vi "Control of Actuator Gait Retraining Actuator Based on IMU Signals.vi"() -> ()   [LabVIEW 2018]
uses:
  <vilib>/Platform/TimedLoop/XDataNode/timing_clust.ctl
  <vilib>/Platform/TimedLoop/XDataNode/nitl_modes.ctl
  <vilib>/Platform/TimedLoop/XDataNode/wakeup.ctl
  <vilib>/DAQmx/write.llb/DAQmx Write (Digital Bool 1Line 1Point).vi
  <vilib>/DAQmx/read.llb/DAQmx Read (Digital Bool 1Line 1Point).vi
  <vilib>/Utility/file.llb/Read Delimited Spreadsheet (DBL).vi
  <vilib>/DAQmx/create/channels.llb/DAQmx Create Channel (DI-Digital Input).vi
  <vilib>/DAQmx/miscellaneous.llb/DAQmx Fill In Error Info.vi
  <vilib>/DAQmx/create/channels.llb/DAQmx Create Channel (DO-Digital Output).vi
  <vilib>/platform/TimedLoop/XDataNode/XDataNode.xnode
  <vilib>/Platform/TimedLoop/XDataNode/XDNodeRunTimeDep.lvlib
  <vilib>/Analysis/NI_AALBase.lvlib
panel:
  out "Stride Pert R":dbl
  out "Stride R T":dbl
  in  "Delay Decimal":dbl
  out "LATENCY MS":dbl
  out "Combined Results":dbl[][][](array[numeric])
  out "INIT END":dbl[][](array[numeric])
  out "Go Right":bool
  out "Go Left":bool
  out "Latency ms":dbl
  out "Stride Pert L":dbl
  out "Stride L T":dbl
  out "EXTEND":bool=TRUE
  out "RETRACT":bool=TRUE
  out "REST":bool=TRUE
  out "MS Start":u32
  out "Boolean":bool=TRUE
  out "Right Stop":dbl
  out "Right Start":dbl
  out "Left Stop":dbl
  out "Left Start":dbl
  out "End L":dbl[](array[numeric])
  out "Init L":dbl[](array[numeric])
  out "End R":dbl[](array[numeric])
  out "Init R":dbl[](array[numeric])
  out "Peaks L":dbl[](array[numeric])
  out "Peaks R":dbl[](array[numeric])
  out "TO R":dbl[](array[numeric])
  out "TO L":dbl[](array[numeric])
  out "Fire Right":bool=TRUE
  out "Fire Left":bool=TRUE
  out "Loop It":i32
  out "x-y":i32
  out "Mu L":dbl
  out "Mu R":dbl
  out "Sig L":dbl format="%0.2f"
  out "Sig R":dbl format="%0.2f"
  out "L Buffer":dbl[](array[numeric])
  out "R Buffer":dbl[](array[numeric])
  out "L Data":dbl[](array[numeric])
  out "R Data":dbl[](array[numeric])
  out "Length L":i32
  out "Swing L":bool
  out "Swing R":bool
  out "Peaked L":bool
  out "Peaked R":bool
  out "Count L":i32=100
  out "Count R":i32=100
  out "Peak Num L":i32=100
  out "Peak Num R":i32=100
  out "TO Num L":i32=100
  out "TO Num R":i32=100
  out "Neg L":i32=100
  out "Neg R":i32=100
  out "Stride L":i32=100
  out "Stride R":i32=100
  out "Stance L":bool
  out "Stance R":bool
  out "Iteration":i32
  out "End":bool=TRUE
  in  "Pressure (Bar)":dbl
  in  "Pert Decimal":dbl
  out "Count":i32
  out "SW2 Off":dbl
  out "transposed array":dbl[][](array[numeric])
  out "Results":dbl[][](array[numeric])
  in  "Extend Time":dbl
  out "Extend Limit":dbl
  out "SW2 Pressed":bool
  in  "V Ext":bool
  in  "V Ret":bool
  out "SW1 Off":dbl
  out "SW1 Pressed":bool
  in  "Extend":bool
  in  "Retract":bool
  out "SW2":bool
  out "SW1":bool
  out "ms passed":dbl
  in  "STOP":bool
  # "May need to switch off if not working"
  # "Percentage of\nGait Cycle"
  # "Percentage of \nGait Cycle"
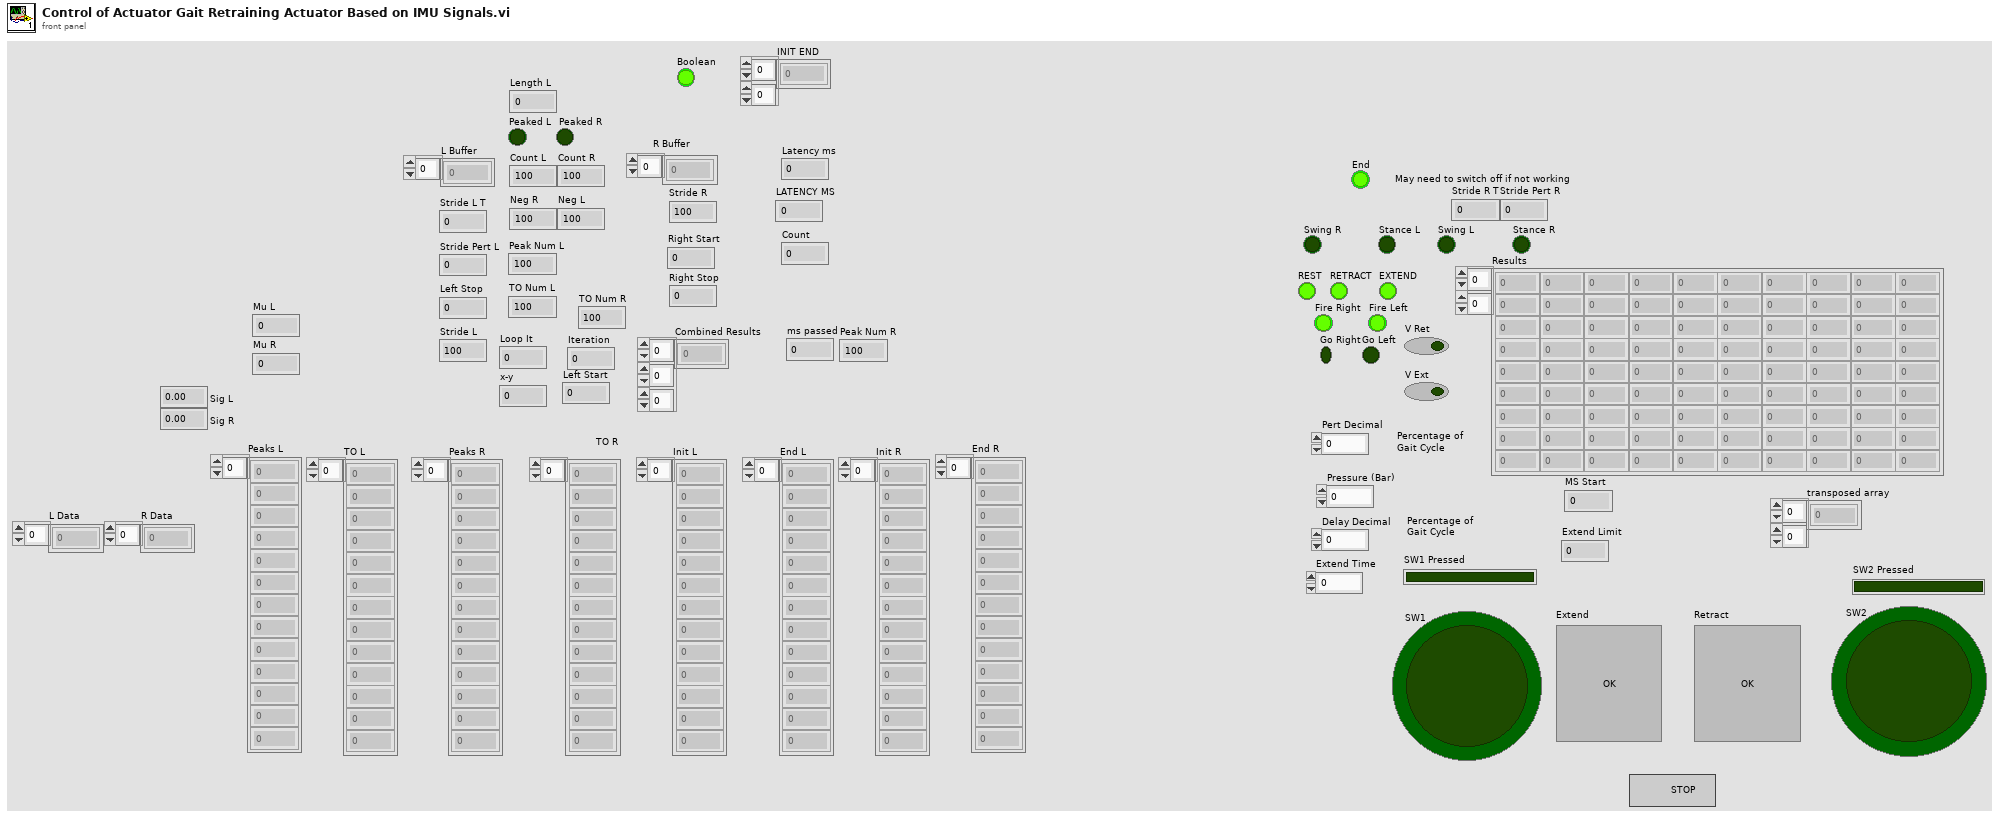
[diagram p1: front panel]
types:
  T1 = typedef "XDNodeRunTimeDep.lvlib/timing_clust.ctl" = cluster{"Expected End [f-1]":u64, "Actual End [f-1]":u64, "Finished Late? [f-1]":bool, "Expected End [i-1]":u64, "Actual End [i-1]":u64, "Finished Late? [i-1]":bool, "Expected Start [i]":u64, "Actual Start [i]":u64, "Expected Start [f]":u64, "Actual Start [f]":u64, "Source Name":string, "Structure Name":string, "Period":i64, "Deadline":i64, "Offset":i64, "Start":i64, "Priority":i32, "Timeout":i32, "Mode":T2, "Wakeup Reason":T3, "Error":errorcluster, "Source Type":string, "Secondary Source Type":string, "Global End Time":u64, "Global Start Time":u64, "Frame Duration":u64, "Iteration Duration":u64, "Assigned CPU":i32, "I/O Scan Engine Mode":u32}
  T2 = typedef "XDNodeRunTimeDep.lvlib/nitl_modes.ctl" = enum32{"No Change", "Process missed periods, maintain original phase", "Discard missed periods, maintain original phase", "Process missed periods, ignore original phase", "Discard missed periods, ignore original phase"}
  T3 = typedef "XDNodeRunTimeDep.lvlib/wakeup.ctl" = enum32{"Normal", "Aborted", "Asynchronous wakeup", "Timing source error", "Timed loop error", "Timeout"}
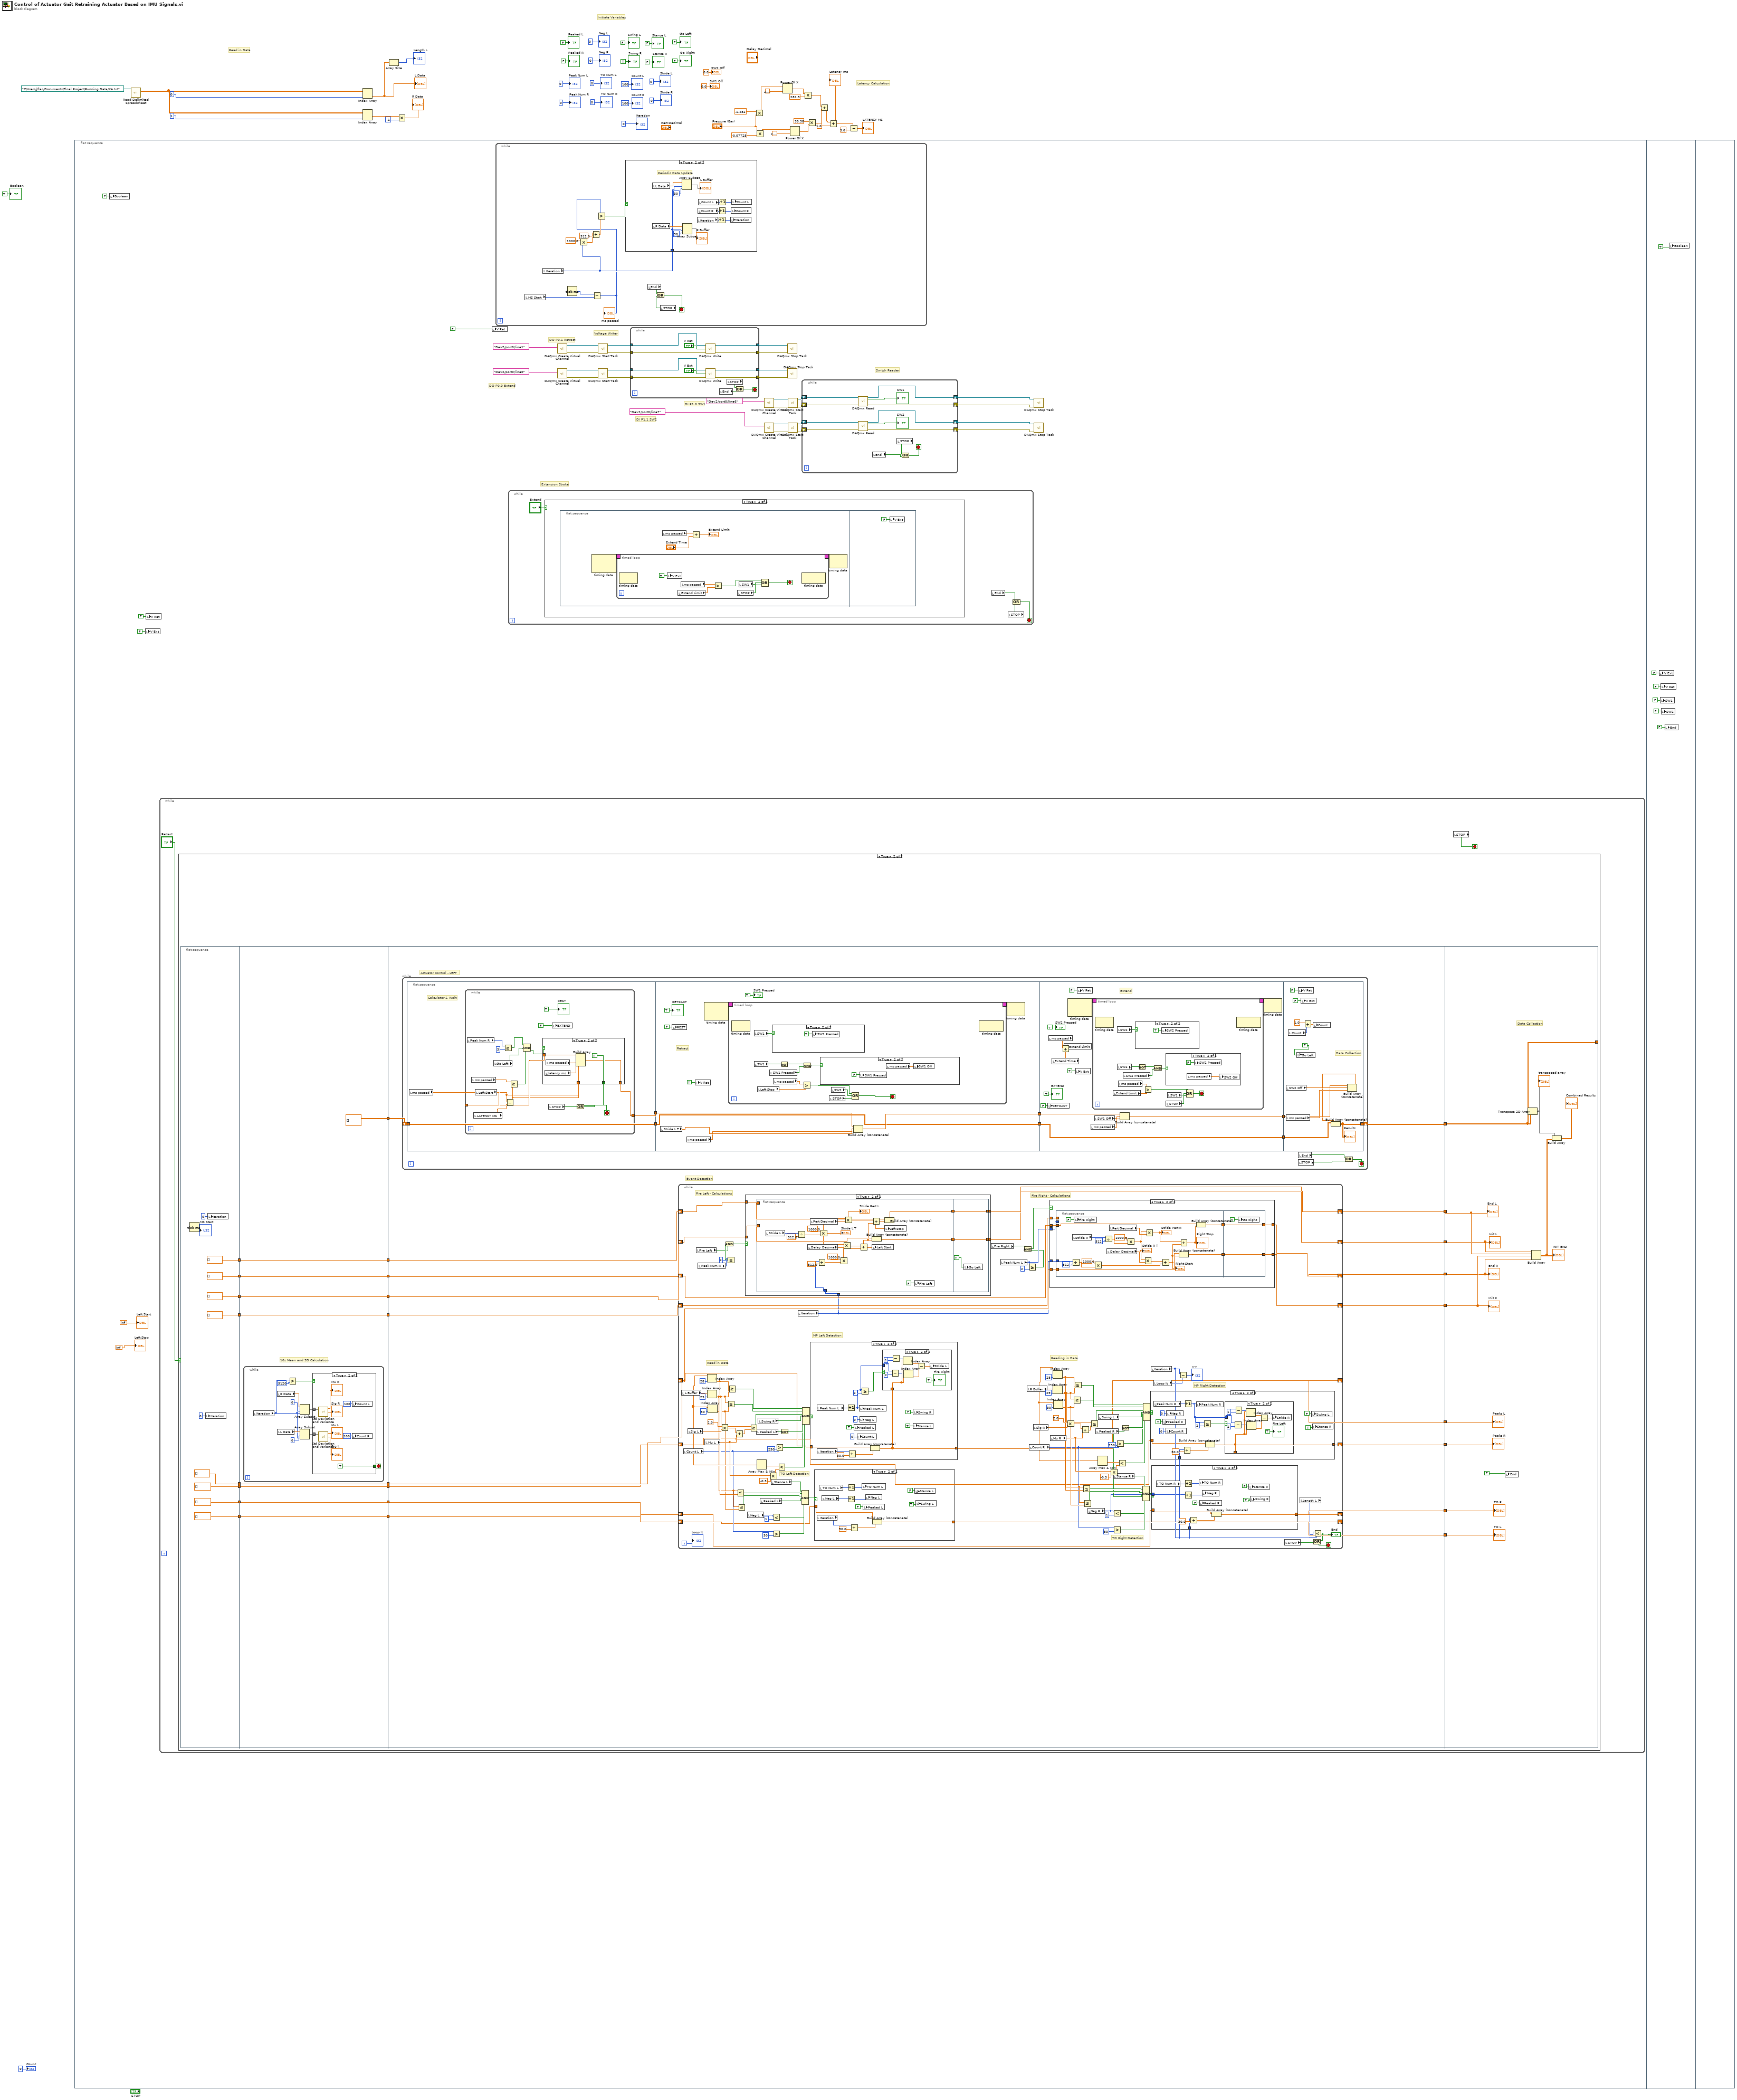
[diagram p0: block diagram]
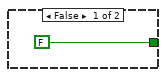
[diagram p4: hidden frame]
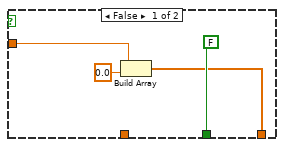
[diagram p5: hidden frame]
diagram:
  # "Latency Calculation"
  # "Initiate Variables"
  # "Read in Data"
  n1 = flat-sequence {
    frame #0 {
      # "Extension Stroke"
      # "Switch Reader"
      # "Voltage Writer"
      # "DO P0.1 Retract"
      # "DO P0.0 Extend"
      # "DI P1.1 SW2"
      # "DI P1.0 SW1"
      n2 = local write "Boolean"(FALSE ("Boolean")) -> ()
      n3 = local write "V Ext"(FALSE ("V Ext")) -> ()
      n4 = local write "V Ret"(FALSE ("V Ret")) -> ()
      n5 = while {
        stop <- w120 stop-if-true
        n6 = case shown="True" "Retract" {
          frame False {
          }
          frame True {
            n7 = flat-sequence {
              tunnel: [dbl[] []] -> w146
              tunnel: [dbl[] []] -> w145
              tunnel: [dbl[] []] -> w144
              tunnel: [dbl[] []] -> w143
              tunnel: [dbl[] []] -> w142
              tunnel: [dbl[] []] -> w141
              tunnel: [dbl[] []] -> w140
              tunnel: [dbl[] []] -> w139
              tunnel: [w166] -> w138
              tunnel: w146 -> [w166]
              tunnel: [w165] -> w137
              tunnel: w145 -> [w165]
              tunnel: [w164] -> w136
              tunnel: w144 -> [w164]
              tunnel: [w163] -> w135
              tunnel: w143 -> [w163]
              tunnel: [w162] -> w134
              tunnel: w142 -> [w162]
              tunnel: [w161] -> w133
              tunnel: w141 -> [w161]
              tunnel: [w160] -> w132
              tunnel: w140 -> [w160]
              tunnel: [w159] -> w131
              tunnel: w139 -> [w159]
              tunnel: [dbl[][] []] -> w121
              tunnel: w138 -> [w204]
              tunnel: w137 -> [w203]
              tunnel: w136 -> [w202]
              tunnel: w135 -> [w201]
              tunnel: w134 -> [w200]
              tunnel: w133 -> [w199]
              tunnel: w132 -> [w198]
              tunnel: w131 -> [w197]
              tunnel: [w196] -> w130
              tunnel: [w195] -> w129
              tunnel: [w194] -> w128
              tunnel: [w193] -> w127
              tunnel: [w192] -> w126
              tunnel: [w191] -> w125
              tunnel: [w190] -> w124
              tunnel: [w189] -> w123
              tunnel: [w188] -> w122
              tunnel: w121 -> [w187]
              tunnel: w130 -> [w576]
              tunnel: w129 -> [w577]
              tunnel: w128 -> [w574]
              tunnel: w127 -> [w575]
              tunnel: w126 -> [w582]
              tunnel: w125 -> [w581]
              tunnel: w124 -> [w580]
              tunnel: w123 -> [w579]
              tunnel: w122 -> [w570]
              tunnel: [w570] -> _
              frame #0 {
                n8 = Tick Count (ms)() -> (millisecond timer value=→"MS Start":u32)
                n9 = local write "Iteration"(0 ("Iteration")) -> ()
                n10 = local write "Iteration"(0 ("Iteration")) -> ()
              }
              frame #1 {
                # "10s Mean and SD Calculation"
                n11 = while {
                  stop <- w167 stop-if-true
                  n12 = local read "Iteration"() -> (w170:i32)
                  n13 = local read "R Data"() -> (w173:dbl[])
                  n14 = local read "L Data"() -> (w174:dbl[])
                  n15 = Greater?(x=w170, y=5120) -> (0:w175:bool)
                  n16 = Array Subset(array=w173, index=0, length=w170) -> (w168:dbl[])
                  n17 = Array Subset(array=w174, index=0, length=w170) -> (w169:dbl[])
                  n18 = case shown="True" w175 {
                    tunnel: w169 -> [_ w186]
                    tunnel: w168 -> [_ w183]
                    tunnel: [FALSE TRUE] -> w167
                    frame False {
                    }
                    frame True {
                      n19 = call <vilib>:"Std Deviation and Variance.vi"("X"=w183) -> ("mean"=→"Mu R":dbl, "standard deviation"=→"Sig R":dbl)  [unwired: 1 in, 1 out]
                      n20 = call <vilib>:"Std Deviation and Variance.vi"("X"=w186) -> ("mean"=→"Mu L":dbl, "standard deviation"=→"Sig L":dbl)  [unwired: 1 in, 1 out]
                      n21 = local write "Count R"(100 ("Count R")) -> ()
                      n22 = local write "Count L"(100 ("Count L")) -> ()
                    }
                  }
                }
              }
              frame #2 {
                # "Actuator Control - LEFT"
                # "Event Detection"
                n23 = while {
                  shift-right: [w208] -> w188
                  shift-left: w187 -> [w209]
                  stop <- w207 stop-if-true
                  n24 = flat-sequence {
                    tunnel: w209 -> [w218]
                    tunnel: [w218] -> w215
                    tunnel: [w217] -> w214
                    tunnel: [w254] -> w213
                    tunnel: [w253] -> w212
                    tunnel: w215 -> [w253]
                    tunnel: w214 -> [w252]
                    tunnel: w213 -> [w286]
                    tunnel: w212 -> [w289]
                    tunnel: [w289] -> w211
                    tunnel: [w282] -> w210
                    tunnel: w211 -> [w310]
                    tunnel: [w318] -> w208
                    tunnel: w210 -> [w314]
                    frame #0 {
                      # "Calculator & Wait"
                      n25 = local read "ms passed"() -> (w216:dbl)
                      n26 = while {
                        tunnel: [w230] -> w217
                        tunnel: w216 -> [w224]
                        stop <- w232 stop-if-true
                        n27 = local read "Peak Num R"() -> (w229:i32)
                        n28 = local read "ms passed"() -> (w222:dbl)
                        n29 = local read "LATENCY MS"() -> (w221:dbl)
                        n30 = local read "Left Start"() -> (w219:dbl)
                        n31 = local read "Go Left"() -> (w226:bool)
                        n32 = Greater Or Equal?(x=w229, y=3) -> (x >= y?=w227:bool)
                        n33 = Subtract(x=w219, y=w221) -> (x-y=w220:dbl)
                        n34 = Greater Or Equal?(x=w222, y=w220) -> (x >= y?=w223:bool)
                        n35 = Compound Arithmetic op=AND(w227, w226, w223) -> (w225:bool)
                        n36 = case shown="True" w225 {
                          tunnel: [FALSE TRUE] -> w231
                          tunnel: w224 -> [w238 w245]
                          tunnel: [w237 w244] -> w230
                          tunnel: w220 -> [_ w241]
                          tunnel: w219 -> [_ w240]
                          frame False {
                            n37 = Build Array(w238, 0.0 ("element")) -> (w237:dbl[])
                          }
                          frame True {
                            n38 = local read "Latency ms"() -> (w242:dbl)
                            n39 = local read "ms passed"() -> (w243:dbl)
                            n40 = Build Array(w245, w243, w242, w241, w240) -> (w244:dbl[])
                          }
                        }
                        n41 = local read "STOP"() -> (w235:bool)
                        n42 = local write "EXTEND"(FALSE ("EXTEND")) -> ()
                        n43 = Or(x=w231, y=w235) -> (x .or. y?=w232:bool)
                        "REST" <- TRUE
                      }
                    }
                    frame #1 {
                      # "Retract"
                      n44 = local read "Stride L T"() -> (w248:dbl)
                      n45 = local write "REST"(FALSE ("REST")) -> ()
                      n46 = local read "ms passed"() -> (w247:dbl)
                      n47 = local write "V Ret"(TRUE ("V Ret")) -> ()
                      n48 = node-c288() -> (w257:T1)  [unwired: 2 in]
                      n49 = timed-loop {
                        timing: w257 -> [_]
                        timing-out: [_] -> w256
                        stop <- w263 stop-if-true
                        n50 = node-c288() -> ()  [unwired: 1 in, 1 out]
                        n51 = local read "SW1"() -> (w258:bool)
                        n52 = local read "SW1"() -> (w261:bool)
                        n53 = local read "Left Stop"() -> (w266:dbl)
                        n54 = local read "SW1 Pressed"() -> (w259:bool)
                        n55 = case shown="True" w258 {
                          frame False {
                          }
                          frame True {
                            n56 = local write "SW1 Pressed"(TRUE ("SW1 Pressed")) -> ()
                          }
                        }
                        n57 = local read "ms passed"() -> (w267:dbl)
                        n58 = Not(x=w261) -> (.not. x?=w260:bool)
                        n59 = Greater?(x=w267, y=w266) -> (0:w265:bool)
                        n60 = And(x=w260, y=w259) -> (x .and. y?=w262:bool)
                        n61 = case shown="True" w262 {
                          frame False {
                          }
                          frame True {
                            n62 = local write "SW1 Pressed"(FALSE ("SW1 Pressed")) -> ()
                            n63 = local read "ms passed"() -> (w270:dbl)
                            n64 = local write "SW1 Off"(w270) -> ()
                          }
                        }
                        n65 = local read "STOP"() -> (w268:bool)
                        n66 = local read "SW2"() -> (w264:bool)
                        n67 = Compound Arithmetic op=OR(w265, w264, w268) -> (w263:bool)
                        n68 = node-c288() -> ()  [unwired: 1 in, 1 out]
                      }
                      n69 = Build Array (concatenate)(w252, w248, w247) -> (w254:dbl[])
                      n70 = node-c288(w256) -> ()  [unwired: 1 out]
                      "SW1 Pressed" <- TRUE ("SW Pressed")
                      "RETRACT" <- TRUE
                    }
                    frame #2 {
                      (unwired) TRUE ("SW Pressed")
                      # "Extend"
                      n71 = local write "RETRACT"(FALSE ("RETRACT")) -> ()
                      n72 = local read "ms passed"() -> (w281:dbl)
                      n73 = local read "Extend Time"() -> (w280:dbl)
                      n74 = Add(x=w281, y=w280) -> (x+y=w279:dbl)
                      n75 = local write "Extend Limit"(w279) -> ()
                      n76 = node-c288() -> (w288:T1)  [unwired: 2 in]
                      n77 = local write "V Ext"(TRUE ("V Ret")) -> ()
                      n78 = local write "V Ret"(FALSE ("V Ret")) -> ()
                      n79 = local read "ms passed"() -> (w284:dbl)
                      n80 = timed-loop {
                        timing: w288 -> [_]
                        timing-out: [_] -> w287
                        stop <- w298 stop-if-true
                        n81 = node-c288() -> ()  [unwired: 1 in, 1 out]
                        n82 = local read "Extend Limit"() -> (w290:dbl)
                        n83 = local read "SW2"() -> (w293:bool)
                        n84 = local read "SW2"() -> (w296:bool)
                        n85 = local read "ms passed"() -> (w292:dbl)
                        n86 = local read "SW2 Pressed"() -> (w294:bool)
                        n87 = case shown="True" w293 {
                          frame False {
                          }
                          frame True {
                            n88 = local write "SW2 Pressed"(TRUE ("SW1 Pressed")) -> ()
                          }
                        }
                        n89 = Not(x=w296) -> (.not. x?=w295:bool)
                        n90 = Greater?(x=w292, y=w290) -> (0:w291:bool)
                        n91 = And(x=w295, y=w294) -> (x .and. y?=w297:bool)
                        n92 = case shown="True" w297 {
                          frame False {
                          }
                          frame True {
                            n93 = local read "ms passed"() -> (w302:dbl)
                            n94 = local write "SW2 Pressed"(FALSE ("SW1 Pressed")) -> ()
                            n95 = local write "SW2 Off"(w302) -> ()
                          }
                        }
                        n96 = local read "STOP"() -> (w300:bool)
                        n97 = local read "SW1"() -> (w299:bool)
                        n98 = Compound Arithmetic op=OR(w291, w299, w300) -> (w298:bool)
                        n99 = node-c288() -> ()  [unwired: 1 in, 1 out]
                      }
                      n100 = local read "SW1 Off"() -> (w283:dbl)
                      n101 = Build Array (concatenate)(w286, w283, w284) -> (w282:dbl[])
                      n102 = node-c288(w287) -> ()  [unwired: 1 out]
                      "EXTEND" <- TRUE
                    }
                    frame #3 {
                      # "Data Collection"
                      n103 = local read "SW2 Off"() -> (w316:dbl)
                      n104 = local read "ms passed"() -> (w315:dbl)
                      n105 = local read "Count"() -> (w311:i32)
                      n106 = local write "Go Left"(FALSE) -> ()
                      n107 = local write "V Ret"(FALSE ("V Ret")) -> ()
                      n108 = local write "V Ext"(FALSE ("V Ext")) -> ()
                      n109 = Add(x=1.0, y=w311) -> (x+y=w312:dbl)
                      n110 = local write "Count"(w312) -> ()
                      n111 = Build Array (concatenate)(w314, w316, w315) -> (w309:dbl[])
                      n112 = Build Array (concatenate)(w310, w309) -> (w318:dbl[][])
                      "Results" <- w318
                    }
                  }
                  n113 = local read "STOP"() -> (w206:bool)
                  n114 = local read "End"() -> (w205:bool)
                  n115 = Compound Arithmetic op=OR(w205, w206) -> (w207:bool)
                }
                n116 = while {
                  shift-right: [w359] -> w192
                  shift-left: w204 -> [w324]
                  shift-right: [w322] -> w191
                  shift-left: w203 -> [w323]
                  shift-right: [w356] -> w189
                  shift-left: w202 -> [w358]
                  shift-right: [w355] -> w190
                  shift-left: w201 -> [w357]
                  shift-right: [w351] -> w196
                  shift-left: w200 -> [w349]
                  shift-right: [w350] -> w195
                  shift-left: w199 -> [w348]
                  shift-right: [w347] -> w194
                  shift-left: w198 -> [w345]
                  shift-right: [w346] -> w193
                  shift-left: w197 -> [w344]
                  i -> [w354]
                  stop <- w327 stop-if-true
                  # "TO Right Detection"
                  # "MP Right Detection"
                  # "Reading in Data"
                  # "TO Left Detection"
                  # "MP Left Detection"
                  # "Read in Data"
                  # "Fire Right - Calculations"
                  # "Fire Left - Calculations"
                  n117 = local read "L Buffer"() -> (w410:dbl[])
                  n118 = local read "Count L"() -> (w397:i32)
                  n119 = local read "Sig L"() -> (w419:dbl)
                  n120 = local read "Fire Left"() -> (w332:bool)
                  n121 = local read "Peak Num R"() -> (w335:i32)
                  n122 = local read "Mu L"() -> (w407:dbl)
                  n123 = Index Array(array=w410, index=28) -> (element=w403:dbl)
                  n124 = Index Array(array=w410, index=29) -> (element=w402:dbl)
                  n125 = Index Array(array=w410, index=30) -> (element=w401:dbl)
                  n126 = Multiply(x=2.0, y=w419) -> (x*y=w418:dbl)
                  n127 = Greater Or Equal?(x=w335, y=2) -> (x >= y?=w333:bool)
                  n128 = And(x=w332, y=w333) -> (x .and. y?=w331:bool)
                  n129 = Greater Or Equal?(x=w402, y=w401) -> (x >= y?=w421:bool)
                  n130 = Greater Or Equal?(x=w402, y=w403) -> (x >= y?=w422:bool)
                  n131 = Add(x=w418, y=w407) -> (x+y=w417:dbl)
                  n132 = Less Or Equal?(x=w402, y=w403) -> (x <= y?=w400:bool)
                  n133 = Less Or Equal?(x=w402, y=w401) -> (x <= y?=w399:bool)
                  n134 = local read "Neg L"() -> (w393:i32)
                  n135 = Greater Or Equal?(x=w402, y=w417) -> (x >= y?=w416:bool)
                  n136 = local read "Peaked L"() -> (w414:bool)
                  n137 = Array Max & Min(array=w410) -> (min value=w409:dbl)  [unwired: 3 out]
                  n138 = local read "Swing R"() -> (w415:bool)
                  n139 = local read "Peaked L"() -> (w398:bool)
                  n140 = Multiply(x=w407, y=-0.3) -> (x*y=w406:dbl)
                  n141 = local read "Stance L"() -> (w343:bool)
                  n142 = Less?(x=w393, y=1) -> (x < y?=w391:bool)
                  n143 = Greater?(x=w397, y=50) -> (0:w395:bool)
                  n144 = Greater?(x=w397, y=250) -> (0:w411:bool)
                  n145 = Less?(x=w409, y=w406) -> (x < y?=w405:bool)
                  n146 = Not(x=w414) -> (.not. x?=w413:bool)
                  n147 = local read "Iteration"() -> (w320:i32)
                  n148 = case shown="True" w331 {
                    tunnel: w349 -> [w462 w468]
                    tunnel: w348 -> [w461 w469]
                    tunnel: [w462 w467] -> w351
                    tunnel: [w461 w466] -> w350
                    tunnel: w320 -> [_ w465]
                    frame False {
                    }
                    frame True {
                      n149 = flat-sequence {
                        tunnel: w469 -> [w490]
                        tunnel: w468 -> [w489]
                        tunnel: w465 -> [w486]
                        tunnel: [w488] -> w464
                        tunnel: [w487] -> w463
                        tunnel: [w492] -> w466
                        tunnel: [w493] -> w467
                        tunnel: w464 -> [w493]
                        tunnel: w463 -> [w492]
                        frame #0 {
                          n150 = local read "Stride L"() -> (w477:i32)
                          n151 = Divide(x=w477, y=512.0) -> (x/y=w479:dbl)
                          n152 = local read "Delay Decimal"() -> (w473:dbl)
                          n153 = local read "Pert Decimal"() -> (w476:dbl)
                          n154 = Divide(x=w486, y=512.0) -> (x/y=w484:dbl)
                          n155 = Multiply(x=1000.0, y=w479) -> (x*y=w474:dbl)
                          "Stride L T" <- w474
                          n156 = Multiply(x=1000.0, y=w484) -> (x*y=w470:dbl)
                          n157 = Multiply(x=w474, y=w473) -> (x*y=w472:dbl)
                          n158 = Multiply(x=w474, y=w476) -> (x*y=w475:dbl)
                          "Stride Pert L" <- w475
                          n159 = Add(x=w472, y=w470) -> (x+y=w471:dbl)
                          n160 = Add(x=w475, y=w471) -> (x+y=w478:dbl)
                          n161 = Build Array (concatenate)(w490, w471) -> (w487:dbl[])
                          n162 = local write "Left Start"(w471) -> ()
                          n163 = Build Array (concatenate)(w489, w478) -> (w488:dbl[])
                          n164 = local write "Left Stop"(w478) -> ()
                          n165 = local write "Fire Left"(FALSE) -> ()
                        }
                        frame #1 {
                          n166 = local write "Go Left"(TRUE) -> ()
                        }
                      }
                    }
                  }
                  n167 = Compound Arithmetic op=AND(w343, w400, w399, w398, w391, w395) -> (w394:bool)
                  n168 = Compound Arithmetic op=AND(w422, w421, w416, w415, w413, w411, w405) -> (w404:bool)
                  n169 = case shown="True" w404 {
                    tunnel: w324 -> [w545 w555]
                    tunnel: [w545 w549] -> w359
                    frame False {
                    }
                    frame True {
                      n170 = local read "Peak Num L"() -> (w559:i32)
                      n171 = local read "Iteration"() -> (w553:i32)
                      n172 = Increment(x=w559) -> (x+1=w548:i32)
                      n173 = Add(x=w553, y=30.0) -> (x+y=w552:dbl)
                      n174 = local write "Peaked L"(TRUE ("Peaked L")) -> ()
                      n175 = local write "Count L"(0 ("Count L")) -> ()
                      n176 = local write "Peak Num L"(w548) -> ()
                      n177 = local write "Neg L"(0 ("Neg L")) -> ()
                      n178 = Greater Or Equal?(x=w548, y=2) -> (x >= y?=w550:bool)
                      n179 = Build Array (concatenate)(w555, w552) -> (w549:dbl[])
                      n180 = case shown="True" w550 {
                        tunnel: w549 -> [_ w569]
                        tunnel: w548 -> [_ w564]
                        frame False {
                        }
                        frame True {
                          n181 = Subtract(x=w564, y=2) -> (x-y=w567:i32)
                          n182 = Subtract(x=w564, y=1) -> (x-y=w562:i32)
                          n183 = Index Array(array=w569, index=w562) -> (element=w566:dbl)
                          n184 = Index Array(array=w569, index=w567) -> (element=w565:dbl)
                          n185 = Subtract(x=w566, y=w565) -> (x-y=w561:dbl)
                          n186 = local write "Stride L"(w561) -> ()
                          "Fire Right" <- TRUE ("Boolean")
                        }
                      }
                      n187 = local write "Stance L"(TRUE ("Stance L")) -> ()
                      n188 = local write "Swing R"(FALSE ("Swing R")) -> ()
                    }
                  }
                  n189 = case shown="True" w394 {
                    tunnel: w358 -> [w532 w537]
                    tunnel: [w532 w535] -> w356
                    frame False {
                    }
                    frame True {
                      n190 = local read "Iteration"() -> (w536:i32)
                      n191 = local read "TO Num L"() -> (w544:i32)
                      n192 = local read "Neg L"() -> (w542:i32)
                      n193 = Increment(x=w544) -> (x+1=w543:i32)
                      n194 = Increment(x=w542) -> (x+1=w541:i32)
                      n195 = Add(x=w536, y=30.0) -> (x+y=w538:dbl)
                      n196 = local write "TO Num L"(w543) -> ()
                      n197 = local write "Peaked L"(FALSE ("Peaked L")) -> ()
                      n198 = local write "Neg L"(w541) -> ()
                      n199 = Build Array (concatenate)(w537, w538) -> (w535:dbl[])
                      n200 = local write "Stance L"(FALSE) -> ()
                      n201 = local write "Swing L"(TRUE) -> ()
                    }
                  }
                  n202 = local read "Fire Right"() -> (w338:bool)
                  n203 = local read "Peak Num L"() -> (w340:i32)
                  n204 = local read "R Buffer"() -> (w321:dbl[])
                  n205 = Greater Or Equal?(x=w340, y=2) -> (x >= y?=w337:bool)
                  n206 = And(x=w338, y=w337) -> (x .and. y?=w336:bool)
                  n207 = local read "Count R"() -> (w365:i32)
                  n208 = local read "Sig R"() -> (w384:dbl)
                  n209 = case shown="True" w336 {
                    tunnel: w345 -> [w427 w435]
                    tunnel: w344 -> [w426 w436]
                    tunnel: [w427 w434] -> w347
                    tunnel: [w426 w428] -> w346
                    tunnel: w340 -> [_ w433]
                    tunnel: w324 -> [_ w432]
                    tunnel: w320 -> [_ w429]
                    frame False {
                    }
                    frame True {
                      n210 = flat-sequence {
                        tunnel: w436 -> [_]
                        tunnel: w435 -> [w457]
                        tunnel: w433 -> [_]
                        tunnel: w432 -> [w440]
                        tunnel: [w456] -> w431
                        tunnel: [w455] -> w430
                        tunnel: w429 -> [w448]
                        tunnel: [w459] -> w428
                        tunnel: [w460] -> w434
                        tunnel: w431 -> [w460]
                        tunnel: w430 -> [w459]
                        frame #0 {
                          n211 = Divide(x=w448, y=512) -> (x/y=w446:dbl)
                          n212 = local read "Stride R"() -> (w453:i32)
                          n213 = local write "Fire Right"(FALSE) -> ()
                          n214 = Multiply(x=1000.0, y=w446) -> (x*y=w441:dbl)
                          n215 = Divide(x=w453, y=512) -> (x/y=w451:dbl)
                          n216 = local read "Delay Decimal"() -> (w444:dbl)
                          n217 = local read "Pert Decimal"() -> (w449:dbl)
                          n218 = Multiply(x=1000.0, y=w451) -> (x*y=w443:dbl)
                          "Stride R T" <- w443
                          n219 = Multiply(x=w443, y=w444) -> (x*y=w442:dbl)
                          n220 = Multiply(x=w443, y=w449) -> (x*y=w439:dbl)
                          "Stride Pert R" <- w439
                          n221 = Add(x=w442, y=w441) -> (x+y=w438:dbl)
                          "Right Start" <- w438
                          n222 = Build Array (concatenate)(w440, w438) -> (w455:dbl[])
                          n223 = Add(x=w439, y=w438) -> (x+y=w437:dbl)
                          "Right Stop" <- w437
                          n224 = Build Array (concatenate)(w457, w437) -> (w456:dbl[])
                        }
                        frame #1 {
                          n225 = local write "Go Right"(TRUE) -> ()
                        }
                      }
                    }
                  }
                  n226 = local read "Mu R"() -> (w374:dbl)
                  n227 = Index Array(array=w321, index=28) -> (element=w370:dbl)
                  n228 = Index Array(array=w321, index=29) -> (element=w369:dbl)
                  n229 = Index Array(array=w321, index=30) -> (element=w368:dbl)
                  n230 = Multiply(x=2.0, y=w384) -> (x*y=w383:dbl)
                  n231 = Greater Or Equal?(x=w369, y=w368) -> (x >= y?=w386:bool)
                  n232 = Greater Or Equal?(x=w369, y=w370) -> (x >= y?=w387:bool)
                  n233 = Add(x=w383, y=w374) -> (x+y=w382:dbl)
                  n234 = Less Or Equal?(x=w369, y=w370) -> (x <= y?=w367:bool)
                  n235 = Less Or Equal?(x=w369, y=w368) -> (x <= y?=w366:bool)
                  n236 = local read "Neg R"() -> (w329:i32)
                  n237 = Greater Or Equal?(x=w369, y=w382) -> (x >= y?=w381:bool)
                  n238 = local read "Peaked R"() -> (w330:bool)
                  n239 = Array Max & Min(array=w321) -> (min value=w376:dbl)  [unwired: 3 out]
                  n240 = local read "Swing L"() -> (w380:bool)
                  n241 = Multiply(x=w374, y=-0.3) -> (x*y=w373:dbl)
                  n242 = Less?(x=w329, y=1) -> (x < y?=w360:bool)
                  n243 = Greater?(x=w365, y=50) -> (0:w363:bool)
                  n244 = local read "Stance R"() -> (w342:bool)
                  n245 = Greater?(x=w365, y=250) -> (0:w377:bool)
                  n246 = Less?(x=w376, y=w373) -> (x < y?=w372:bool)
                  n247 = Not(x=w330) -> (.not. x?=w379:bool)
                  n248 = Compound Arithmetic op=AND(w342, w367, w366, w330, w360, w363) -> (w362:bool)
                  n249 = Compound Arithmetic op=AND(w387, w386, w381, w380, w379, w377, w372) -> (w371:bool)
                  n250 = local read "Iteration"() -> (w328:i32)
                  n251 = case shown="True" w371 {
                    tunnel: w323 -> [w507 w515]
                    tunnel: [w507 w514] -> w322
                    tunnel: w328 -> [_ w508]
                    frame False {
                    }
                    frame True {
                      n252 = local read "Peak Num R"() -> (w521:i32)
                      n253 = local write "Peaked R"(TRUE ("Peaked L")) -> ()
                      n254 = local write "Count R"(0 ("Count L")) -> ()
                      n255 = local write "Neg R"(0 ("Neg L")) -> ()
                      n256 = Add(x=w508, y=30.0) -> (x+y=w516:dbl)
                      n257 = Increment(x=w521) -> (x+1=w513:i32)
                      n258 = local write "Peak Num R"(w513) -> ()
                      n259 = Greater Or Equal?(x=w513, y=2) -> (x >= y?=w511:bool)
                      n260 = Build Array (concatenate)(w515, w516) -> (w514:dbl[])
                      n261 = case shown="True" w511 {
                        tunnel: w514 -> [_ w531]
                        tunnel: w513 -> [_ w526]
                        frame False {
                        }
                        frame True {
                          n262 = Subtract(x=w526, y=2) -> (x-y=w529:i32)
                          n263 = Subtract(x=w526, y=1) -> (x-y=w524:i32)
                          n264 = Index Array(array=w531, index=w524) -> (element=w528:dbl)
                          n265 = Index Array(array=w531, index=w529) -> (element=w527:dbl)
                          n266 = Subtract(x=w528, y=w527) -> (x-y=w523:dbl)
                          n267 = local write "Stride R"(w523) -> ()
                          "Fire Left" <- TRUE
                        }
                      }
                      n268 = local write "Swing L"(FALSE) -> ()
                      n269 = local write "Stance R"(TRUE) -> ()
                    }
                  }
                  n270 = case shown="True" w362 {
                    tunnel: w357 -> [w494 w500]
                    tunnel: [w494 w499] -> w355
                    tunnel: w329 -> [_ w496]
                    tunnel: w328 -> [_ w495]
                    frame False {
                    }
                    frame True {
                      n271 = local read "TO Num R"() -> (w506:i32)
                      n272 = Increment(x=w506) -> (x+1=w505:i32)
                      n273 = Increment(x=w496) -> (x+1=w504:i32)
                      n274 = Add(x=w495, y=30.0) -> (x+y=w501:dbl)
                      n275 = local write "TO Num R"(w505) -> ()
                      n276 = local write "Peaked R"(FALSE ("Peaked L")) -> ()
                      n277 = local write "Neg R"(w504) -> ()
                      n278 = Build Array (concatenate)(w500, w501) -> (w499:dbl[])
                      n279 = local write "Stance R"(FALSE) -> ()
                      n280 = local write "Swing R"(TRUE) -> ()
                    }
                  }
                  n281 = local read "Loop It"() -> (w353:i32)
                  n282 = Subtract(x=w328, y=w353) -> (x-y=→"x-y":i32)
                  n283 = local read "STOP"() -> (w325:bool)
                  n284 = local read "Length L"() -> (w341:i32)
                  n285 = Less?(x=w341, y=w328) -> (x < y?=w326:bool)
                  "End" <- w326
                  n286 = Or(x=w326, y=w325) -> (x .or. y?=w327:bool)
                  "Loop It" <- w354
                }
              }
              frame #3 {
                # "Data Collection"
                n287 = local write "End"(FALSE) -> ()
                n288 = Transpose 2D Array(2D array=w570) -> (transposed array=w572:dbl[][])
                "transposed array" <- w572
                n289 = Build Array(w577, w576, w575, w574) -> (w573:dbl[][])
                "INIT END" <- w573
                n290 = Build Array(w572, w573) -> (→"Combined Results":dbl[][][])
                "End L" <- w576
                "Init L" <- w577
                "End R" <- w574
                "Init R" <- w575
                "Peaks L" <- w582
                "Peaks R" <- w581
                "TO R" <- w580
                "TO L" <- w579
              }
            }
          }
        }
        n291 = local read "STOP"() -> (w120:bool)
      }
      n292 = local write "V Ret"(FALSE ("V Ret")) -> ()
      n293 = while {
        stop <- w603 stop-if-true
        n294 = local read "MS Start"() -> (w606:u32)
        n295 = local read "Iteration"() -> (w598:i32)
        n296 = Tick Count (ms)() -> (millisecond timer value=w607:u32)
        n297 = Multiply(x=1000.0, y=w598) -> (x*y=w600:dbl)
        n298 = Divide(x=w600, y=512.0) -> (x/y=w602:dbl)
        n299 = Subtract(x=w607, y=w606) -> (x-y=w596:u32)
        "ms passed" <- w596
        n300 = Greater?(x=w596, y=w602) -> (0:w597:bool)
        n301 = case shown="True" w597 {
          tunnel: w598 -> [_ w610]
          frame False {
          }
          frame True {
            # "Periodic Data Update"
            n302 = local read "L Data"() -> (w618:dbl[])
            n303 = local read "R Data"() -> (w616:dbl[])
            n304 = Array Subset(array=w618, index=w610, length=30) -> (→"L Buffer":dbl[])
            n305 = Array Subset(array=w616, index=w610, length=30) -> (→"R Buffer":dbl[])
            n306 = local read "Iteration"() -> (w608:i32)
            n307 = local read "Count R"() -> (w613:i32)
            n308 = local read "Count L"() -> (w614:i32)
            n309 = Increment(x=w608) -> (x+1=w609:i32)
            n310 = Increment(x=w613) -> (x+1=w611:i32)
            n311 = Increment(x=w614) -> (x+1=w612:i32)
            n312 = local write "Iteration"(w609) -> ()
            n313 = local write "Count R"(w611) -> ()
            n314 = local write "Count L"(w612) -> ()
          }
        }
        n315 = local read "End"() -> (w605:bool)
        n316 = local read "STOP"() -> (w604:bool)
        n317 = Compound Arithmetic op=OR(w605, w604) -> (w603:bool)
      }
      n318 = while {
        stop <- w85 stop-if-true
        n319 = case shown="True" "Extend" {
          frame False {
          }
          frame True {
            n320 = flat-sequence {
              frame #0 {
                n321 = node-c288() -> (w93:T1)  [unwired: 2 in]
                n322 = timed-loop {
                  timing: w93 -> [_]
                  timing-out: [_] -> w92
                  stop <- w95 stop-if-true
                  n323 = node-c288() -> ()  [unwired: 1 in, 1 out]
                  n324 = local write "V Ext"(TRUE ("V Ext")) -> ()
                  n325 = local read "Extend Limit"() -> (w98:dbl)
                  n326 = local read "ms passed"() -> (w99:dbl)
                  n327 = Greater?(x=w99, y=w98) -> (0:w97:bool)
                  n328 = local read "STOP"() -> (w100:bool)
                  n329 = local read "SW1"() -> (w96:bool)
                  n330 = Compound Arithmetic op=OR(w97, w96, w100) -> (w95:bool)
                  n331 = node-c288() -> ()  [unwired: 1 in, 1 out]
                }
                n332 = local read "ms passed"() -> (w89:dbl)
                n333 = Add(x=w89, y="Extend Time") -> (x+y=→"Extend Limit":dbl)
                n334 = node-c288(w92) -> ()  [unwired: 1 out]
              }
              frame #1 {
                n335 = local write "V Ext"(FALSE ("V Ext")) -> ()
              }
            }
          }
        }
        n336 = local read "End"() -> (w87:bool)
        n337 = local read "STOP"() -> (w86:bool)
        n338 = Compound Arithmetic op=OR(w87, w86) -> (w85:bool)
      }
      n339 = call-poly <vilib>:"DAQmx Create Virtual Channel.vi"("lines"=tag "Dev2/port0/line1") -> ("task out"=w66:refnum<k21>, "error out"=w65:errorcluster)  [unwired: 13 in]
      n340 = call-poly <vilib>:"DAQmx Create Virtual Channel.vi"("lines"=tag "Dev2/port0/line0") -> ("task out"=w69:refnum<k21>, "error out"=w70:errorcluster)  [unwired: 13 in]
      n341 = call <vilib>:"DAQmx Start Task.vi"("task/channels in"=w66, "error in"=w65) -> ("task out"=w64:refnum<k21>, "error out"=w63:errorcluster)  [unwired: 12 in]
      n342 = call <vilib>:"DAQmx Start Task.vi"("task/channels in"=w69, "error in"=w70) -> ("task out"=w62:refnum<k21>, "error out"=w61:errorcluster)  [unwired: 12 in]
      n343 = while {
        tunnel: w64 -> [w118]
        tunnel: w63 -> [w117]
        tunnel: w62 -> [w116]
        tunnel: w61 -> [w115]
        tunnel: [w112] -> w60
        tunnel: [w111] -> w59
        tunnel: [w110] -> w58
        tunnel: [w109] -> w57
        stop <- w106 stop-if-true
        n344 = call-poly <vilib>:"DAQmx Write.vi"("task/channels in"=w118, "data"="V Ret", "error in"=w117) -> ("task out"=w112:refnum<k21>, "error out"=w111:errorcluster)  [unwired: 10 in, 1 out]
        n345 = call-poly <vilib>:"DAQmx Write.vi"("task/channels in"=w116, "data"="V Ext", "error in"=w115) -> ("task out"=w110:refnum<k21>, "error out"=w109:errorcluster)  [unwired: 10 in, 1 out]
        n346 = local read "End"() -> (w107:bool)
        n347 = local read "STOP"() -> (w108:bool)
        n348 = Compound Arithmetic op=OR(w108, w107) -> (w106:bool)
      }
      n349 = call-poly <vilib>:"DAQmx Create Virtual Channel.vi"("lines"=tag "Dev2/port0/line6") -> ("task out"=w82:refnum<k21>, "error out"=w83:errorcluster)  [unwired: 13 in]
      n350 = call-poly <vilib>:"DAQmx Create Virtual Channel.vi"("lines"=tag "Dev2/port0/line7") -> ("task out"=w81:refnum<k21>, "error out"=w80:errorcluster)  [unwired: 13 in]
      n351 = call <vilib>:"DAQmx Stop Task.vi"("task/channels in"=w60, "error in"=w59) -> ()  [unwired: 12 in, 2 out]
      n352 = call <vilib>:"DAQmx Stop Task.vi"("task/channels in"=w58, "error in"=w57) -> ()  [unwired: 12 in, 2 out]
      n353 = call <vilib>:"DAQmx Start Task.vi"("task/channels in"=w82, "error in"=w83) -> ("task out"=w78:refnum<k21>, "error out"=w77:errorcluster)  [unwired: 12 in]
      n354 = call <vilib>:"DAQmx Start Task.vi"("task/channels in"=w81, "error in"=w80) -> ("task out"=w76:refnum<k21>, "error out"=w75:errorcluster)  [unwired: 12 in]
      n355 = while {
        shift-right: [w591] -> w74
        shift-left: w78 -> [w595]
        shift-right: [w590] -> w73
        shift-left: w77 -> [w594]
        shift-right: [w589] -> w72
        shift-left: w76 -> [w593]
        shift-right: [w588] -> w71
        shift-left: w75 -> [w592]
        stop <- w583 stop-if-true
        n356 = call-poly <vilib>:"DAQmx Read.vi"("task/channels in"=w595, "error in"=w594) -> ("task out"=w591:refnum<k21>, "data"=→"SW1":bool, "error out"=w590:errorcluster)  [unwired: 11 in]
        n357 = call-poly <vilib>:"DAQmx Read.vi"("task/channels in"=w593, "error in"=w592) -> ("task out"=w589:refnum<k21>, "data"=→"SW2":bool, "error out"=w588:errorcluster)  [unwired: 11 in]
        n358 = local read "End"() -> (w584:bool)
        n359 = local read "STOP"() -> (w585:bool)
        n360 = Compound Arithmetic op=OR(w585, w584) -> (w583:bool)
      }
      n361 = call <vilib>:"DAQmx Stop Task.vi"("task/channels in"=w74, "error in"=w73) -> ()  [unwired: 12 in, 2 out]
      n362 = call <vilib>:"DAQmx Stop Task.vi"("task/channels in"=w72, "error in"=w71) -> ()  [unwired: 12 in, 2 out]
      "Left Stop" <- inf
      "Left Start" <- inf
    }
    frame #1 {
      n363 = local write "V Ext"(FALSE ("V Ext")) -> ()
      n364 = local write "SW1"(FALSE ("SW1")) -> ()
      n365 = local write "V Ret"(FALSE ("V Ret")) -> ()
      n366 = local write "SW2"(FALSE ("SW2")) -> ()
      n367 = local write "End"(FALSE ("End")) -> ()
      n368 = local write "Boolean"(TRUE) -> ()
    }
    frame #2 {
    }
  }
  n369 = call-poly <vilib>:"Read Delimited Spreadsheet.vi"("file path (dialog if empty)"=path "C:/Users/jflac/Documents/Final Project/Running Data/XA.txt") -> ("all rows"=w26:dbl[][])  [unwired: 9 in, 5 out]
  n370 = Index Array(array=w26, index (col)=0 ("disabled index (col)")) -> (element=w31:dbl[])  [unwired: 1 in]
  "L Data" <- w31
  n371 = Index Array(array=w26, index (col)=1 ("disabled index (col)")) -> (element=w28:dbl[])  [unwired: 1 in]
  n372 = Array Size(array=w31) -> (size(s)=→"Length L":i32)
  n373 = Multiply(x=w28, y=-1) -> (x*y=→"R Data":dbl[])
  n374 = Multiply(x=-1.482, y="Pressure (Bar)") -> (x*y=w16:dbl)
  n375 = Multiply(x="Pressure (Bar)", y=-0.07725) -> (x*y=w14:dbl)
  n376 = Power Of X(1:2.718281828459045, 2:w16) -> (0:w13:dbl)
  n377 = Power Of X(1:2.718281828459045, 2:w14) -> (0:w12:dbl)
  n378 = Multiply(x=w13, y=281.5) -> (x*y=w9:dbl)
  n379 = Multiply(x=35.38, y=w12) -> (x*y=w8:dbl)
  n380 = Add(x=w9, y=w8) -> (x+y=w5:dbl)
  n381 = Add(x=w5, y=1.0) -> (x+y=w3:dbl)
  "Latency ms" <- w3
  n382 = Subtract(x=w3, y=3.0) -> (x-y=→"LATENCY MS":dbl)
  "Count" <- 0
  "Swing L" <- FALSE
  "Swing R" <- TRUE
  "Peaked L" <- FALSE
  "Peaked R" <- FALSE
  "Count L" <- 100
  "Count R" <- 100
  "Peak Num L" <- 0
  "Peak Num R" <- 0
  "TO Num L" <- 0
  "TO Num R" <- 0
  "Neg L" <- 0
  "Neg R" <- 0
  "Stride L" <- 0
  "Stride R" <- 0
  "Stance L" <- FALSE
  "Stance R" <- FALSE
  "Iteration" <- 0
  "SW2 Off" <- 0.0 ("SW2 Off")
  "SW1 Off" <- 0.0 ("SW1 Off")
  "Boolean" <- TRUE ("Boolean")
  "Go Left" <- FALSE
  "Go Right" <- FALSE
